vi "Load Last Config.vi"(8 "error in (no error)":errorcluster) -> (0 "error out":errorcluster, 2 "Process Settings.lvclass":refnum<class "Process Settings.lvclass">, 3 "All Hardware":refnum<class "Hardware Settings.lvclass">)   [LabVIEW 2017]
uses:
  Hardware Settings/Hardware Settings.lvclass
  Process Settings/Process Settings.lvclass
  Process Settings/Process Settings.lvclass/Process Settings.ctl
  Process Settings/Accessors/Read Hardware Settings.vi
  <vilib>/Utility/config.llb/Read Key (String).vi
  <vilib>/Utility/config.llb/NI_LVConfig.lvlib
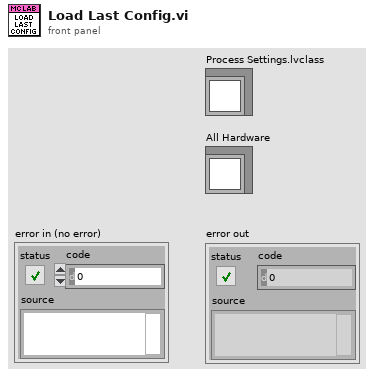
[diagram p1: front panel]
types:
  T1 = typedef "NI_LVConfig.lvlib/Config Data RefNum.ctl" = refnum<k1>
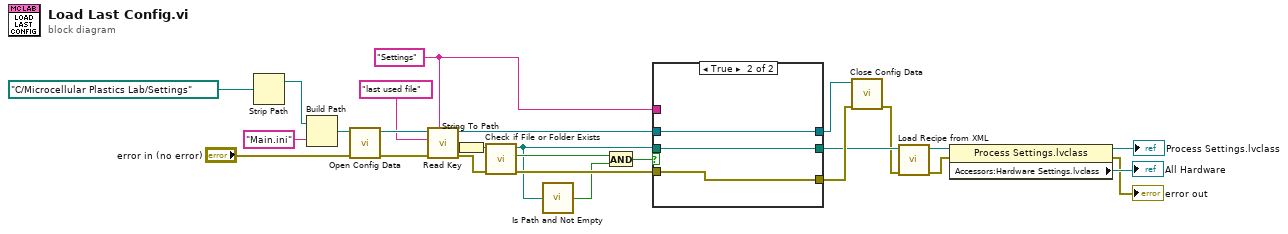
[diagram p0: block diagram]
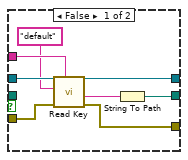
[diagram p2: hidden frame]
diagram:
  w16 = "Settings" ("key")
  n1 = Strip Path(path=path "C:/Microcellular Plastics Lab/Settings" ("Path")) -> (stripped path=w26:path)  [unwired: 1 out]
  n2 = Build Path(base path=w26, name or relative path="Main.ini") -> (appended path=w24:path)
  n3 = call <vilib>:"Open Config Data.vi"("error in (no error)"="error in (no error)", "configuration file path"=w24) -> ("error out"=w22:errorcluster, "refnum"=w23:T1)  [unwired: 7 in, 1 out]
  n4 = call-poly <vilib>:"Read Key.vi"("section"=w16, "error in (no error)"=w22, "key"="last used file", "refnum"=w23) -> ("error out"=w18:errorcluster, "value"=w19:string, "refnum out"=w20:T1)  [unwired: 4 in, 1 out]
  n5 = String To Path(string=w19) -> (path=w6:path)
  n6 = call <vilib>:"Check if File or Folder Exists.vi"("error in (no error)"=w18, "path"=w6) -> ("error out"=w17:errorcluster, "file or folder exists?"=w4:bool, "dup path"=w2:path)  [unwired: 7 in]
  n7 = call <vilib>:"Is Path and Not Empty.vi"("path"=w2) -> ("Is Path and Not Empty?"=w5:bool)  [unwired: 4 in]
  n8 = And(x=w4, y=w5) -> (x .and. y?=w3:bool)
  n9 = case shown="True" w3 {
    tunnel: w20 -> [w35 w36]
    tunnel: w16 -> [w34 _]
    tunnel: [w32 w38] -> w15
    tunnel: w17 -> [w31 w38]
    tunnel: [w28 w37] -> w13
    tunnel: w2 -> [_ w37]
    tunnel: [w29 w36] -> w14
    frame False {
      n10 = call-poly <vilib>:"Read Key.vi"("section"=w34, "error in (no error)"=w31, "key"="default", "refnum"=w35) -> ("error out"=w32:errorcluster, "value"=w30:string, "refnum out"=w29:T1)  [unwired: 4 in, 1 out]
      n11 = String To Path(string=w30) -> (path=w28:path)
    }
    frame True {
    }
  }
  n12 = call <vilib>:"Close Config Data.vi"("error in (no error)"=w15, "refnum"=w14) -> ("error out"=w12:errorcluster)  [unwired: 8 in, 1 out]
  n13 = call "Load Recipe from XML.vi"("error in (no error)"=w12, "Path"=w13) -> ("error out"=w10:errorcluster, "Selected Recipe Settings"=w8:refnum<class "Process Settings.lvclass">)  [unwired: 8 in]
  n14 = property class="Process Settings.lvclass"(reference=w8, error in=w10) -> (reference out=→"Process Settings.lvclass":refnum<class "Process Settings.lvclass">, error out=→"error out":errorcluster, "Accessors:Hardware Settings.lvclass"=→"All Hardware":refnum<class "Hardware Settings.lvclass">)
